vi "MCAST string to TDMS path.vi"(11 "MCAST path":string) -> (3 "TDMS path":path)   [LabVIEW 2013]
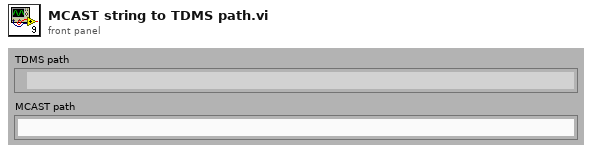
[diagram p1: front panel]
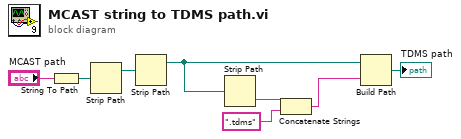
[diagram p0: block diagram]
diagram:
  n1 = String To Path(string="MCAST path") -> (path=w8:path)
  n2 = Strip Path(path=w8) -> (stripped path=w2:path)  [unwired: 1 out]
  n3 = Strip Path(path=w2) -> (stripped path=w1:path)  [unwired: 1 out]
  n4 = Strip Path(path=w1) -> (name=w6:string)  [unwired: 1 out]
  n5 = Concatenate Strings(w6, ".tdms" ("string")) -> (w4:string)
  n6 = Build Path(base path=w1, name or relative path=w4) -> (appended path=→"TDMS path":path)
